vi "GetCollisionParams.vi"(8 "error in (no error)":errorcluster, 11 "Pong in":refnum<class "Pong.lvclass">) -> (0 "error out":errorcluster, 1 "UpDownLeftRightCollide":bool[](array[boolean]), 2 "UpDownLeftRightBounce":dbl[](array[numeric]), 3 "Pong out":refnum<class "Pong.lvclass">)   [LabVIEW 2019, in "RT_Game.lvlib" / "Pong.lvclass"]
uses:
  Pong.lvclass
  C:/Users/FreshBob/Dropbox/VIs/myRIO_GameConsole/RT/RT_Game/Game/Game.lvclass
  Menu/States.ctl
  Game/Game.lvclass/Game.ctl
  Game/Read State.vi
  Game/Game.lvclass
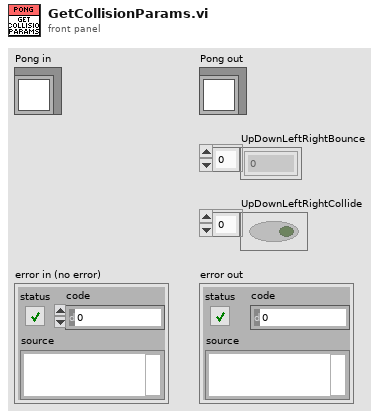
[diagram p1: front panel]
types:
  T1 = typedef "RT_Game.lvlib/Game.lvclass/States.ctl" = enum16{"Init", "Restart", "Menu", "Game", "Resume", "ToggleSingleplayer", "LoadNextGame", "ExitToMenu", "NewHighscore", "GameOver", "SlideOut"}
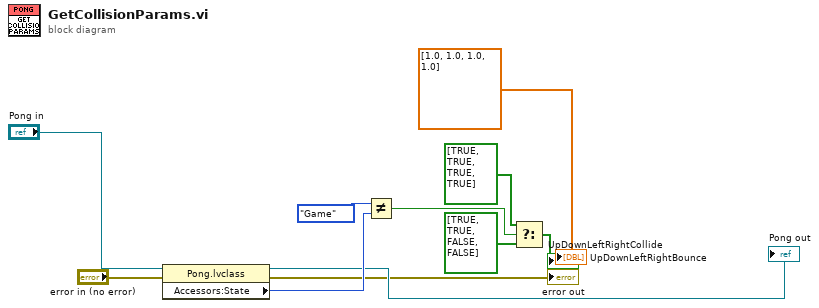
[diagram p0: block diagram]
diagram:
  n1 = property class="Pong.lvclass"(reference="Pong in", error in="error in (no error)") -> (reference out=→"Pong out":refnum<class "Pong.lvclass">, error out=→"error out":errorcluster, "Accessors:State"=w11:T1)
  n2 = Not Equal?(x=States."Game" ("y"), y=w11) -> (x != y?=w5:bool)
  n3 = Select(t=bool[] [TRUE, TRUE, TRUE, TRUE] ("UpDownLeftRightCollide"), s=w5, f=bool[] [TRUE, TRUE, FALSE, FALSE] ("UpDownLeftRightCollide")) -> (s? t:f=→"UpDownLeftRightCollide":bool[])
  "UpDownLeftRightBounce" <- dbl[] [1.0, 1.0, 1.0, 1.0] ("UpDownLeftRightBounce")
